vi "dfd_Calculate Decimation Output Len.vi"(4 "factor":i32, 6 "output phase":i32, 7 "current phase":i32, 10 "signal in len":i32) -> (2 "signal out len":i32)   [LabVIEW 2017, in "NI_DigFilter_FXP.lvlib"]
uses:
  <vilib>/addons/Digital Filter Design/NI_DigFilter_FXP.lvlib
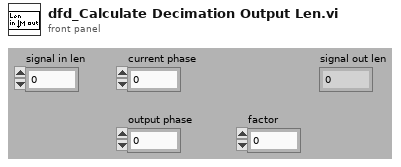
[diagram p1: front panel]
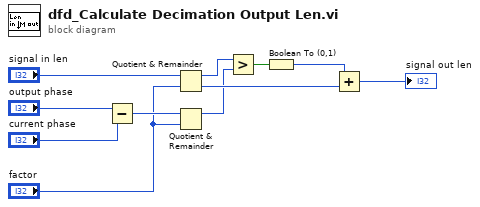
[diagram p0: block diagram]
diagram:
  n1 = Subtract(x="output phase", y="current phase") -> (x-y=w9:i32)
  n2 = Quotient & Remainder(x="signal in len", y="factor") -> (x-y*floor(x/y)=w4:i32, floor(x/y)=w5:i32)
  n3 = Quotient & Remainder(x=w9, y="factor") -> (x-y*floor(x/y)=w3:i32)  [unwired: 1 out]
  n4 = Greater?(x=w4, y=w3) -> (0:w2:bool)
  n5 = Boolean To (0,1)(Boolean=w2) -> (0, 1=w11:i16)
  n6 = Add(x=w11, y=w5) -> (x+y=→"signal out len":i32)
